vi "AnalogDeadzone.vi"(9 "Input 3":dbl, 10 "Input 2":dbl, 11 "Input":dbl) -> (1 "Output 3":dbl, 2 "Output 2":dbl, 3 "Output":dbl)   [LabVIEW 2014]
panel:
  out "Output 6":dbl
  out "Output 5":dbl
  out "Output 4":dbl
  in  "Input 6":dbl
  in  "Input 5":dbl
  in  "Input 4":dbl
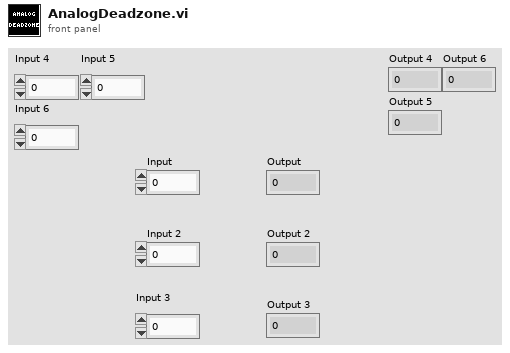
[diagram p1: front panel]
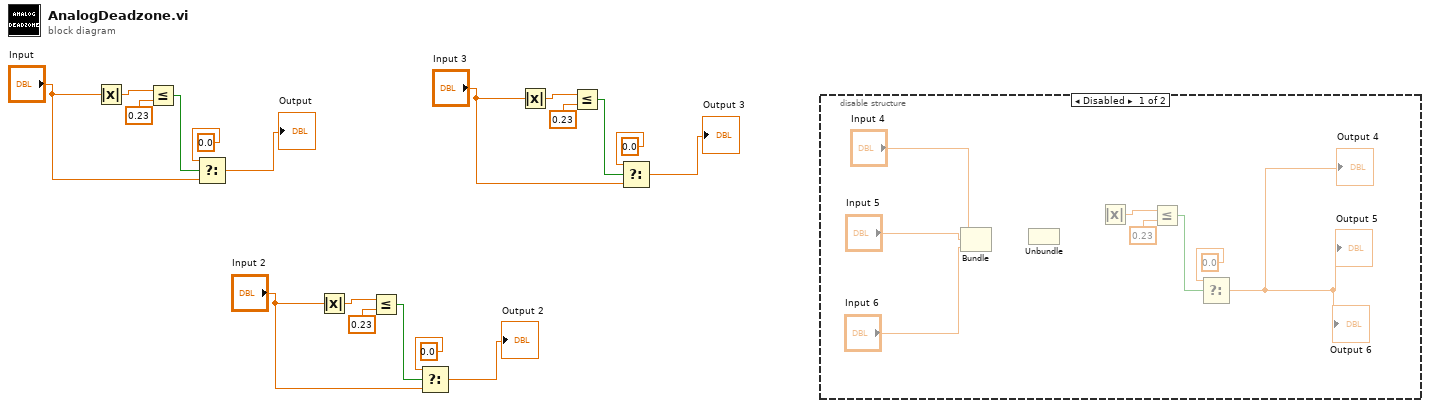
[diagram p0: block diagram]
diagram:
  n1 = Absolute Value(x="Input") -> (abs(x)=w18:dbl)
  n2 = Less Or Equal?(x=w18, y=0.23) -> (x <= y?=w16:bool)
  n3 = Select(t=0.0, s=w16, f="Input") -> (s? t:f=→"Output":dbl)
  n4 = Absolute Value(x="Input 2") -> (abs(x)=w12:dbl)
  n5 = Less Or Equal?(x=w12, y=0.23) -> (x <= y?=w10:bool)
  n6 = Select(t=0.0, s=w10, f="Input 2") -> (s? t:f=→"Output 2":dbl)
  n7 = Absolute Value(x="Input 3") -> (abs(x)=w6:dbl)
  n8 = Less Or Equal?(x=w6, y=0.23) -> (x <= y?=w4:bool)
  n9 = Select(t=0.0, s=w4, f="Input 3") -> (s? t:f=→"Output 3":dbl)
  n10 = disable-structure shown="Disabled" {
    frame Disabled {
      n11 = Bundle("Input 4"="Input 4", "Input 5"="Input 5", "Input 6"="Input 6") -> ()  [unwired: 1 in, 1 out]
      n12 = Unbundle() -> ()  [unwired: 1 in, 2 out]
      n13 = Absolute Value() -> (abs(x)=w23:dbl)  [unwired: 1 in]
      n14 = Less Or Equal?(x=w23, y=0.23) -> (x <= y?=w21:bool)
      n15 = Select(t=0.0, s=w21) -> (s? t:f=→"Output 4" →"Output 5" →"Output 6":dbl)  [unwired: 1 in]
    }
    frame Enabled {
    }
  }
